vi "csv.vi"(4 "deney no":string, 5 "1D data":dbl[](array[numeric]), 6 "Table Control":string[][](table), 7 "2D data":dbl[][](array[numeric]), 8 "Boolean-String":bool, 9 "Boolean-Namber":bool, 10 "Boolean-Namber 1D":bool, 11 "base path":path) -> (0 "appended path":path, 1 "error strng":errorcluster, 2 "error num":errorcluster, 3 "error 1D":errorcluster)   [LabVIEW 2020]
uses:
  <vilib>/Utility/sysdir.llb/System Directory Type.ctl
  <vilib>/Utility/file.llb/Write Delimited Spreadsheet (string).vi
  <vilib>/Utility/file.llb/Write Delimited Spreadsheet (DBL).vi
panel:
  out "Adres":path
  out "Çıktı2":string[][](table)
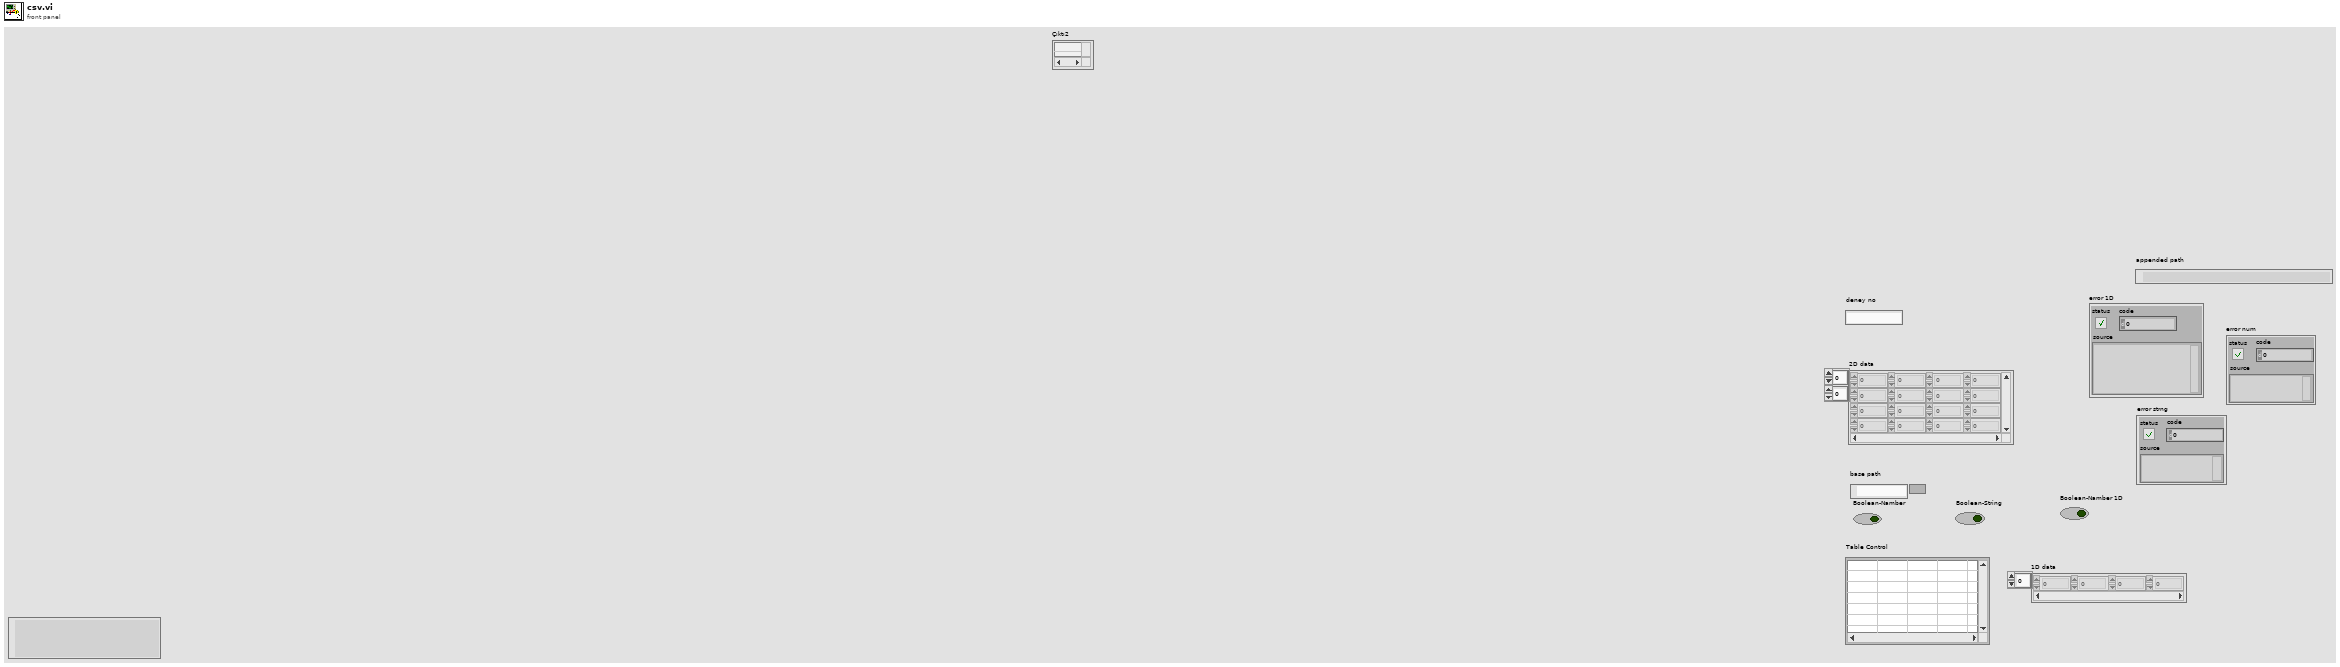
[diagram p1: front panel]
types:
  T1 = typedef "System Directory Type.ctl" = i32
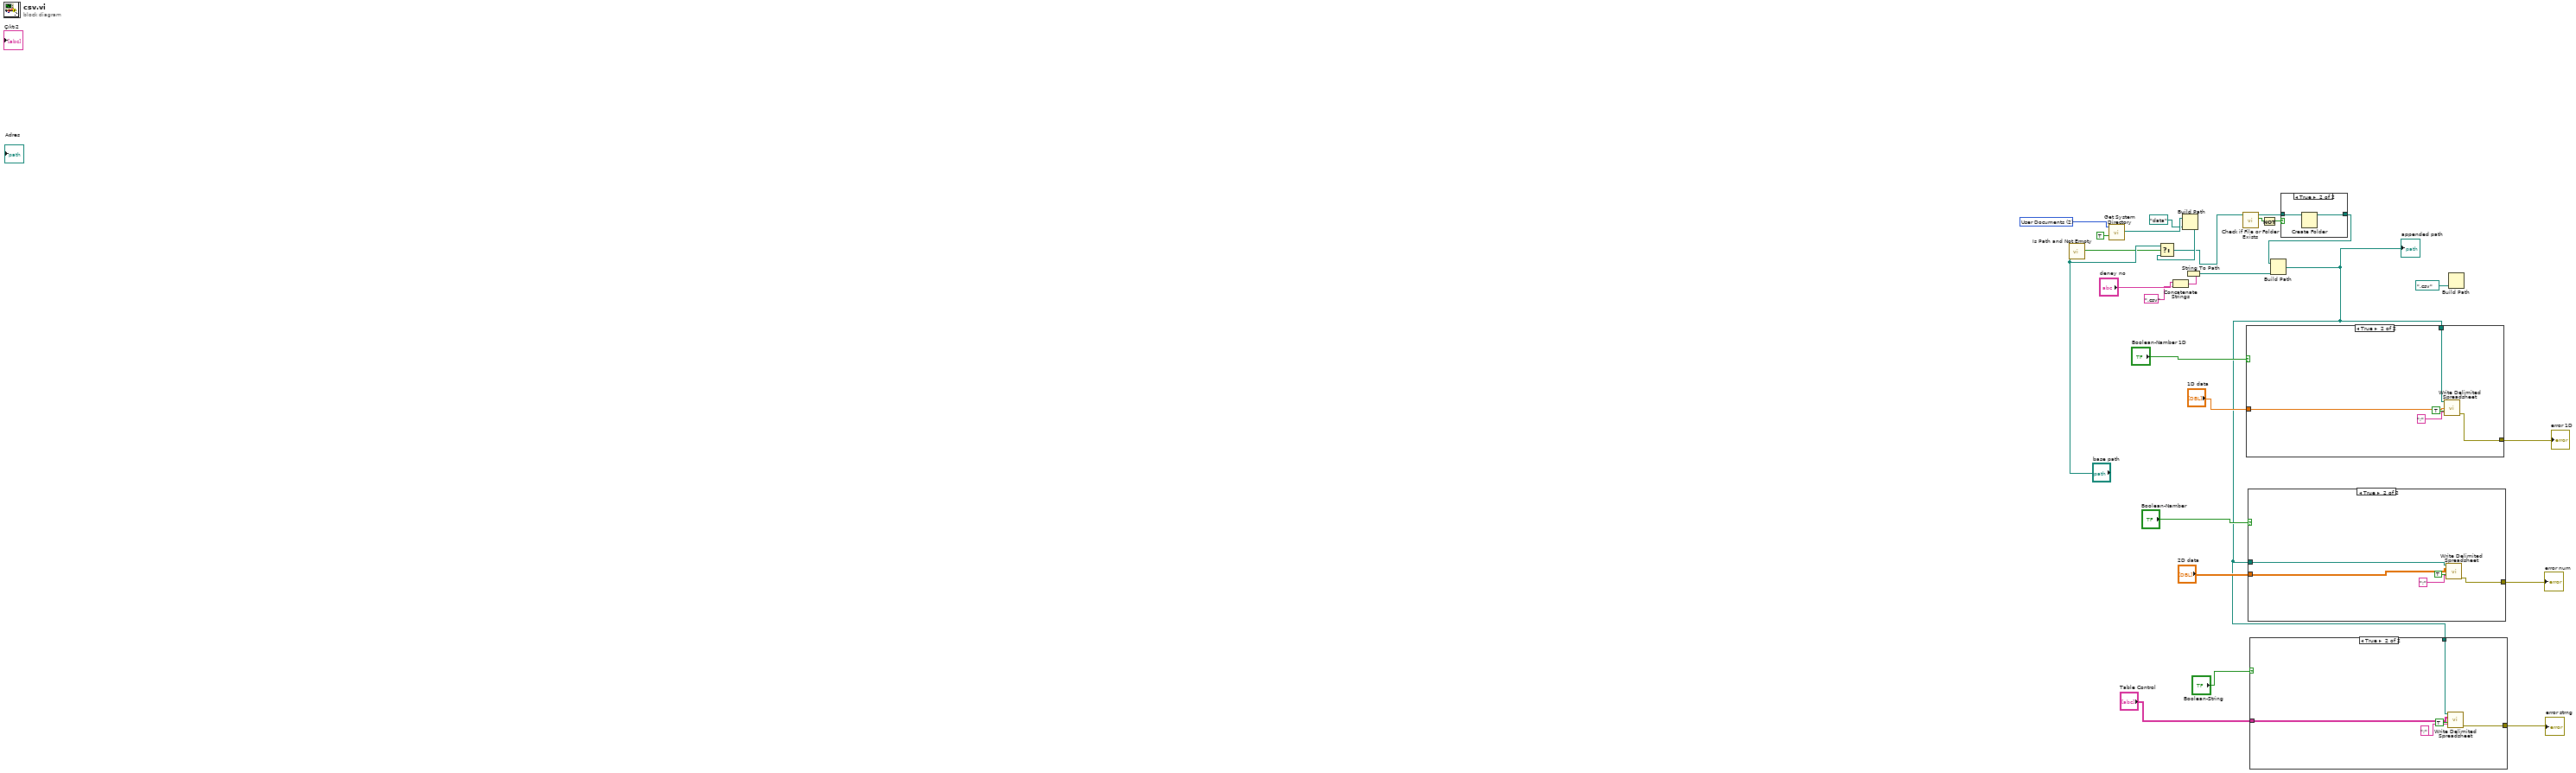
[diagram p0: block diagram]
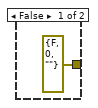
[diagram p3: hidden frame]
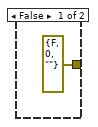
[diagram p4: hidden frame]
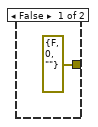
[diagram p5: hidden frame]
diagram:
  w15 = T1 2 items=["User Home"=0, "User Desktop"=1, "User Documents"=2, "User Application Data"=3, "User Preferences"=4, "User Temporary"=5, "Public Documents"=6, "Public Application Data"=7, "Public Preferences"=8, "Public Cache"=13, "System Core Libraries"=9, "System Installed Libraries"=10, "Application Files"=11, "Boot Volume Root"=12] ("system directory type")
  n1 = call <vilib>:"Is Path and Not Empty.vi"("path"="base path") -> ("Is Path and Not Empty?"=w17:bool)  [unwired: 4 in]
  n2 = call <vilib>:"Get System Directory.vi"("create directory if not found? (F)"=TRUE, "system directory type"=w15) -> ("system directory"=w11:path)  [unwired: 9 in]
  n3 = Concatenate Strings("deney no", ".csv" ("string")) -> (w5:string)
  n4 = Build Path(base path=w11, name or relative path=path "data") -> (appended path=w9:path)
  n5 = Select(t="base path", s=w17, f=w9) -> (s? t:f=w3:path)
  n6 = String To Path(string=w5) -> (path=w4:path)
  n7 = call <vilib>:"Check if File or Folder Exists.vi"("path"=w3) -> ("file or folder exists?"=w12:bool, "dup path"=w14:path)  [unwired: 8 in, 1 out]
  n8 = Not(x=w12) -> (.not. x?=w13:bool)
  n9 = case shown="True" w13 {
    tunnel: [w28 w29] -> w2
    tunnel: w14 -> [w28 w30]
    frame False {
    }
    frame True {
      n10 = Create Folder(path (use dialog)=w30) -> (created path=w29:path)  [unwired: 2 in, 2 out]
    }
  }
  n11 = Build Path(base path=w2, name or relative path=w4) -> (appended path=w1:path)
  "appended path" <- w1
  n12 = case shown="True" "Boolean-Namber 1D" {
    tunnel: "1D data" -> [_ w35]
    tunnel: [errorcluster {"status"=FALSE, "code"=0, "source"=""} ("error out") w34] -> w20
    tunnel: w1 -> [_ w33]
    frame False {
    }
    frame True {
      n13 = call-poly <vilib>:"Write Delimited Spreadsheet.vi"("file path (dialog if empty)"=w33, "1D data"=w35, "append to file? (new file:F)"=TRUE, "delimiter (\\t)"=";" ("delimiter (\\t)")) -> ("error out"=w34:errorcluster)  [unwired: 10 in, 1 out]
    }
  }
  "error 1D" <- w20
  n14 = case shown="True" "Boolean-Namber" {
    tunnel: "2D data" -> [_ w41]
    tunnel: [errorcluster {"status"=FALSE, "code"=0, "source"=""} ("error out") w40] -> w19
    tunnel: w1 -> [_ w39]
    frame False {
    }
    frame True {
      n15 = call-poly <vilib>:"Write Delimited Spreadsheet.vi"("file path (dialog if empty)"=w39, "2D data"=w41, "append to file? (new file:F)"=TRUE, "delimiter (\\t)"=";" ("delimiter (\\t)")) -> ("error out"=w40:errorcluster)  [unwired: 10 in, 1 out]
    }
  }
  "error num" <- w19
  n16 = case shown="True" "Boolean-String" {
    tunnel: "Table Control" -> [_ w47]
    tunnel: [errorcluster {"status"=FALSE, "code"=0, "source"=""} ("error out") w46] -> w18
    tunnel: w1 -> [_ w45]
    frame False {
    }
    frame True {
      n17 = call-poly <vilib>:"Write Delimited Spreadsheet.vi"("file path (dialog if empty)"=w45, "2D data"=w47, "append to file? (new file:F)"=TRUE, "delimiter (\\t)"=";" ("delimiter (\\t)")) -> ("error out"=w46:errorcluster)  [unwired: 10 in, 1 out]
    }
  }
  "error strng" <- w18
  n18 = Build Path(name or relative path=path ".csv") -> ()  [unwired: 1 in, 1 out]
